vi "GDFsaveEventTableToCSV.vi"(8 "error in":errorcluster, 11 "GDFv1.x.lvclass in":refnum<class "GDFv1.x.lvclass">) -> (0 "error out":errorcluster, 3 "GDFv1.x.lvclass out":refnum<class "GDFv1.x.lvclass">)   [LabVIEW 2016, in "GDF File Reader.lvlib" / "GDFv1.x.lvclass"]
uses:
  GDFv1.x.lvclass
  GDFv1.x.lvclass/GDFv1.x.ctl
panel:
  # "This VI is a part of BCI Design library, http://www.ru-bci.org \nCopyright © 2020, Sotnikov Peter, All rights reserved. License: CC BY-NC 4.0"
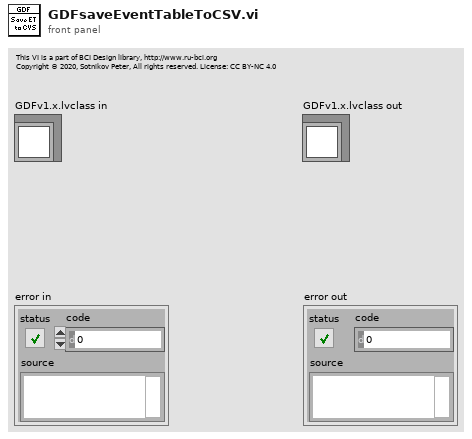
[diagram p1: front panel]
types:
  T1 = enum16{"open", "replace", "create", "open or create", "replace or create", "replace or create with confirmation"}
  T2 = typedef "GDF File Reader.lvlib/EventDataType.ctl" = cluster{"Position (in samples)":u32, "EventType":string, "Channel":u16, "Duration (in samples)":u32}
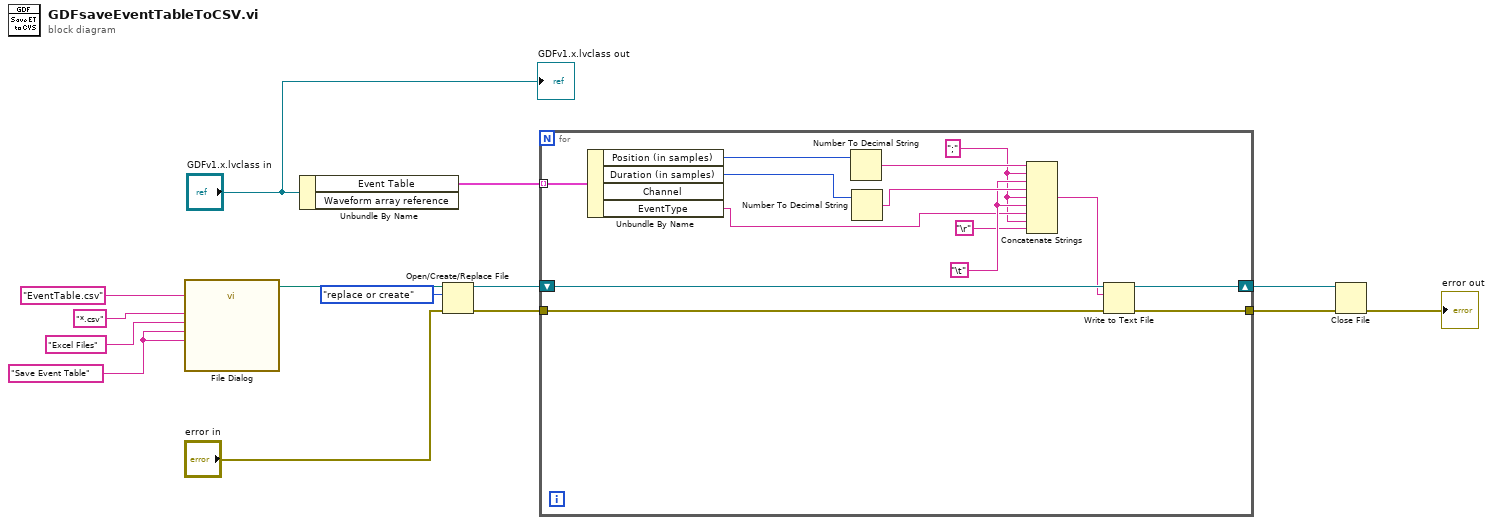
[diagram p0: block diagram]
diagram:
  w9 = "Save Event Table" ("button label")
  n1 = call "File Dialog"("prompt"=w9, "button label"=w9, "default name"="EventTable.csv", "pattern (all files)"="*.csv", "pattern label"="Excel Files") -> ("selected path"=w8:path)  [unwired: 7 in, 3 out]
  n2 = Unbundle By Name("GDFv1.x.lvclass in") -> ("Event Table"=w13:T2[])  [unwired: 1 out]
  n3 = Open/Create/Replace File(file path (use dialog)=w8, error in="error in", operation (0:open)=T1."replace or create") -> (refnum out=w5:refnum<file>, error out=w6:errorcluster)  [unwired: 3 in, 1 out]
  n4 = for {
    tunnel: w13 -> [w28] mode=indexing
    tunnel: w6 -> [w22]
    shift-right: [w26] -> w2
    shift-left: w5 -> [w27]
    tunnel: [w21] -> w3
    w16 = ";" ("string")
    w18 = "\t"
    n5 = Unbundle By Name(w28) -> ("Position (in samples)"=w25:u32, "Duration (in samples)"=w24:u32, "EventType"=w17:string)  [unwired: 1 out]
    n6 = Number To Decimal String(number=w25) -> (decimal integer string=w20:string)  [unwired: 1 in]
    n7 = Number To Decimal String(number=w24) -> (decimal integer string=w19:string)  [unwired: 1 in]
    n8 = Concatenate Strings(w20, w16, w18, w19, w16, w18, w17, w16, "\r") -> (w23:string)
    n9 = Write to Text File(file (use dialog)=w27, text=w23, error in=w22) -> (refnum out=w26:refnum<file>, error out=w21:errorcluster)  [unwired: 1 in, 1 out]
  }
  n10 = Close File(refnum=w2, error in=w3) -> (error out=→"error out":errorcluster)  [unwired: 1 out]
  "GDFv1.x.lvclass out" <- "GDFv1.x.lvclass in"
